vi "Kroki Plot.vi"(8 "error in":errorcluster, 11 "Render String":string) -> (0 "error out":errorcluster, 2 "image data":T1, 3 "Kroki Plot":picture)   [LabVIEW 2020, in "SimpleDependencyInspector.lvlib"]
uses:
  SimpleDependencyInspector.lvlib
  <vilib>/picture/picture.llb/imagedata.ctl
  <vilib>/httpClient/POSTBuffer.vi
  <vilib>/wsapi/NI_WebServices.lvlib
  <vilib>/httpClient/LabVIEWHTTPClient.lvlib
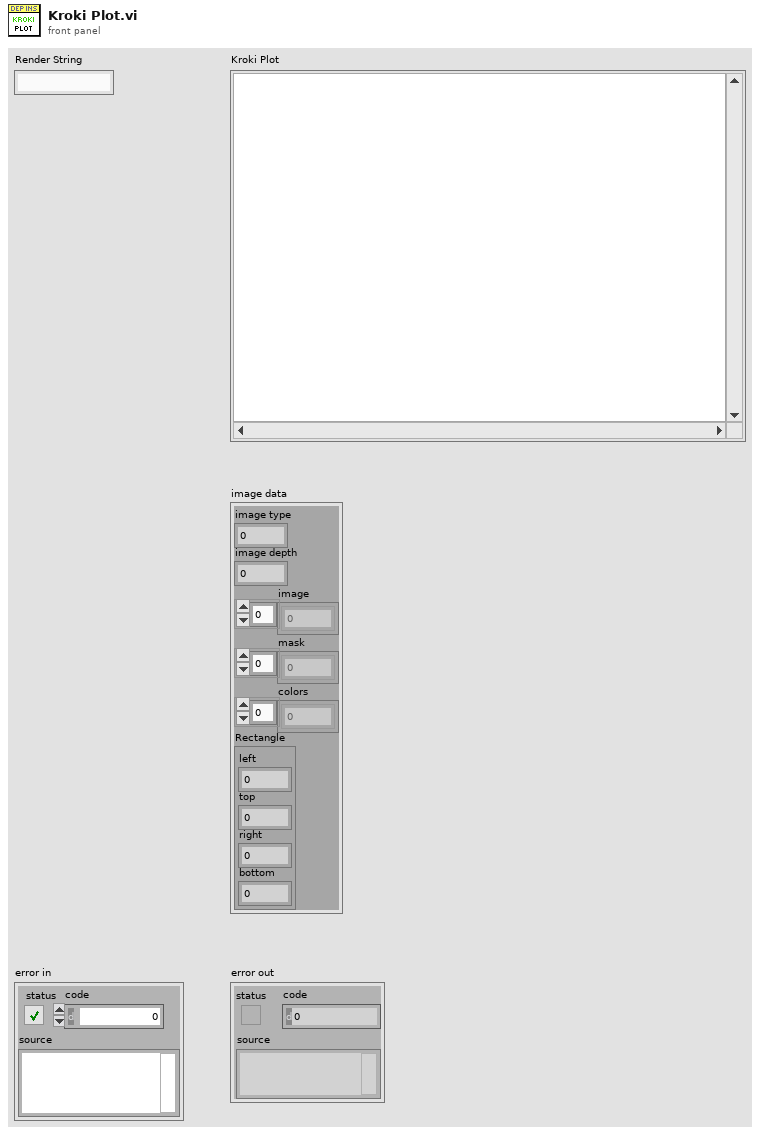
[diagram p1: front panel]
types:
  T1 = typedef "imagedata.ctl" = cluster{"image type":i32, "image depth":i32, "image":u8[], "mask":u8[], "colors":u32[], "Rectangle":cluster{"left":i16, "top":i16, "right":i16, "bottom":i16}}
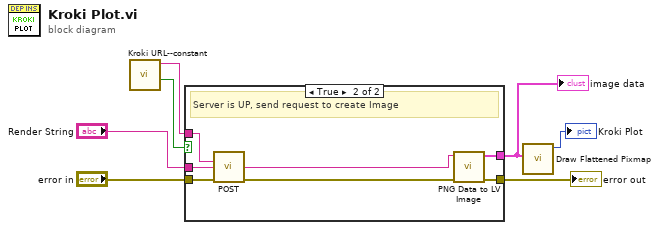
[diagram p0: block diagram]
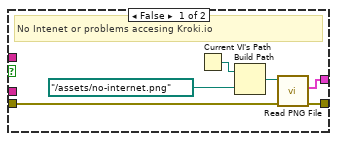
[diagram p2: hidden frame]
diagram:
  n1 = call "Kroki URL--constant.vi"() -> ("Server is UP"=w4:bool, "Kroki Full URL"=w5:string)  [unwired: 9 in, 1 out]
  n2 = case shown="True" w4 {
    tunnel: "error in" -> [w13 w19]
    tunnel: [w12 w18] -> w6
    tunnel: w5 -> [_ w16]
    tunnel: [w8 w15] -> w3
    tunnel: "Render String" -> [_ w14]
    frame False {
      # "No Intenet or problems accesing Kroki.io"
      n3 = Current VI's Path() -> (path=w10:path)
      n4 = Build Path(base path=w10, name or relative path=path "../assets/no-internet.png") -> (appended path=w9:path)
      n5 = call <vilib>:"Read PNG File.vi"("error in (no error)"=w13, "path to PNG file"=w9) -> ("error out"=w12:errorcluster, "image data"=w8:T1)  [unwired: 7 in, 1 out]
    }
    frame True {
      # "Server is UP, send request to create Image"
      n6 = call-poly <vilib>:"POST.vi"("url"=w16, "buffer"=w14, "error in (no error)"=w19) -> ("body"=w17:string, "error out"=w20:errorcluster)  [unwired: 9 in, 2 out]
      n7 = call <vilib>:"PNG Data to LV Image.vi"("error in (no error)"=w20, "png data"=w17) -> ("error out"=w18:errorcluster, "image data"=w15:T1)  [unwired: 8 in]
    }
  }
  "error out" <- w6
  "image data" <- w3
  n8 = call <vilib>:"Draw Flattened Pixmap.vi"("image data"=w3) -> ("new picture"=→"Kroki Plot":picture)  [unwired: 8 in]
